vi "CreateOrderSlip.vi"(8 "error in (no error)":errorcluster, 11 "PizzaTestDrive in":refnum<class "PizzaTestDrive.lvclass">) -> (0 "error out":errorcluster, 2 "OrderSlip":T1[](array[typedef]), 3 "PizzaTestDrive out":refnum<class "PizzaTestDrive.lvclass">)   [LabVIEW 2020]
uses:
  PizzaTestDrive.lvclass
  PizzaStore/PizzaStore.lvclass
  OrderPizza.ctl
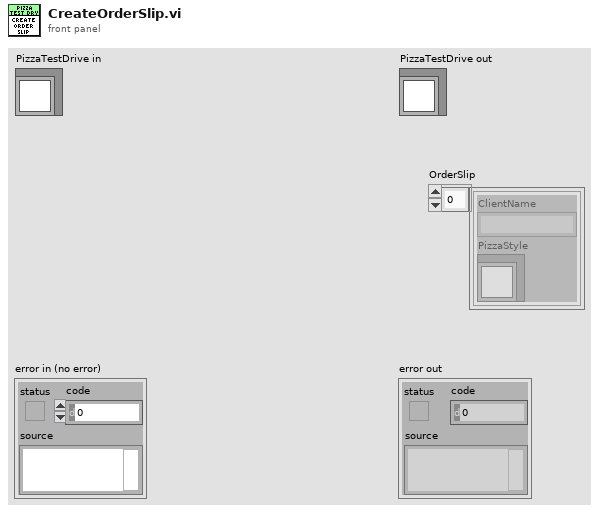
[diagram p1: front panel]
types:
  T1 = typedef "OrderPizza.ctl" = cluster{"ClientName":string, "PizzaStyle":refnum<class "PizzaStore.lvclass">}
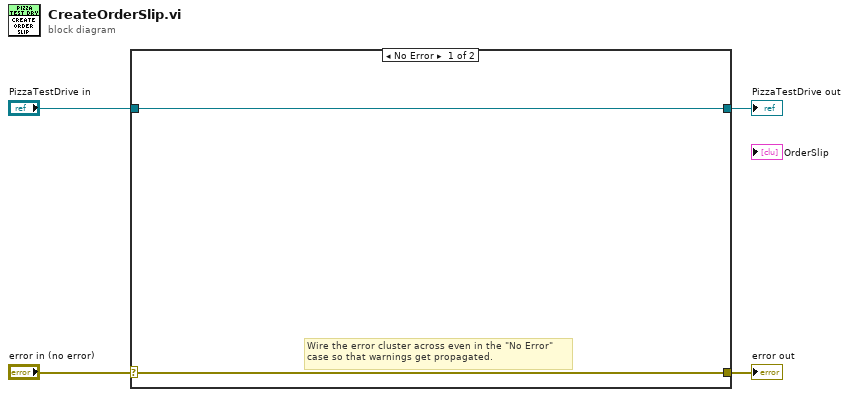
[diagram p0: block diagram]
diagram:
  n1 = case shown="No Error" "error in (no error)" {
    selector: "error in (no error)" -> [w5 w8]
    tunnel: [w5 w8] -> w3
    tunnel: [w6 w7] -> w1
    tunnel: "PizzaTestDrive in" -> [w6 w7]
    frame No Error {
      # "Wire the error cluster across even in the \"No Error\"\ncase so that warnings get propagated."
    }
    frame Error {
    }
  }
  "error out" <- w3
  "PizzaTestDrive out" <- w1
